vi "Main UI.vi"() -> ()   [LabVIEW 2014]
doc: "This template is for the Queued Message Handler design pattern.\n\nThe Event Handling Loop generates messages based on user interface actions.\n\nThe Message Handling Loop processes messages generated by the Event Handling Loop, or by other messages. The messages are string values, so new messages can be added easily to the Message Cases case structure in the Message Handling Loop. Each message cluster can also provide an optional value for Message Data, which is a variant that can be converted to whatever message-specific data is required."
uses:
  controls/UI Data.ctl
  support/Message Queue/Message Queue.lvlib
  support/User Event - Stop/User Event - Stop.lvlib
panel:
  out "DNL_Data Display <Replace Me>":string
  in  "DNL_Do Something Else <Replace Me>":bool
  in  "DNL_Do Something <Replace Me>":bool
  in  "DNL_Stop Button":bool
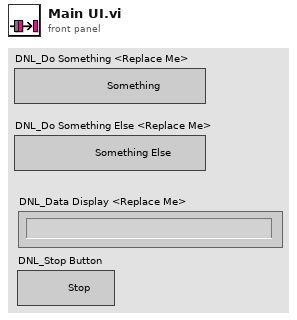
[diagram p1: front panel]
types:
  T1 = typedef "UI Data.ctl" = cluster{"DNL_Boolean <Replace Me>":bool, "DNL_String <Replace Me>":string, "DNL_Numeric <Replace Me>":dbl}
  T2 = typedef "Message Queue.lvlib/All Message Queues.ctl" = cluster{"DNL_UI":refnum<queue>}
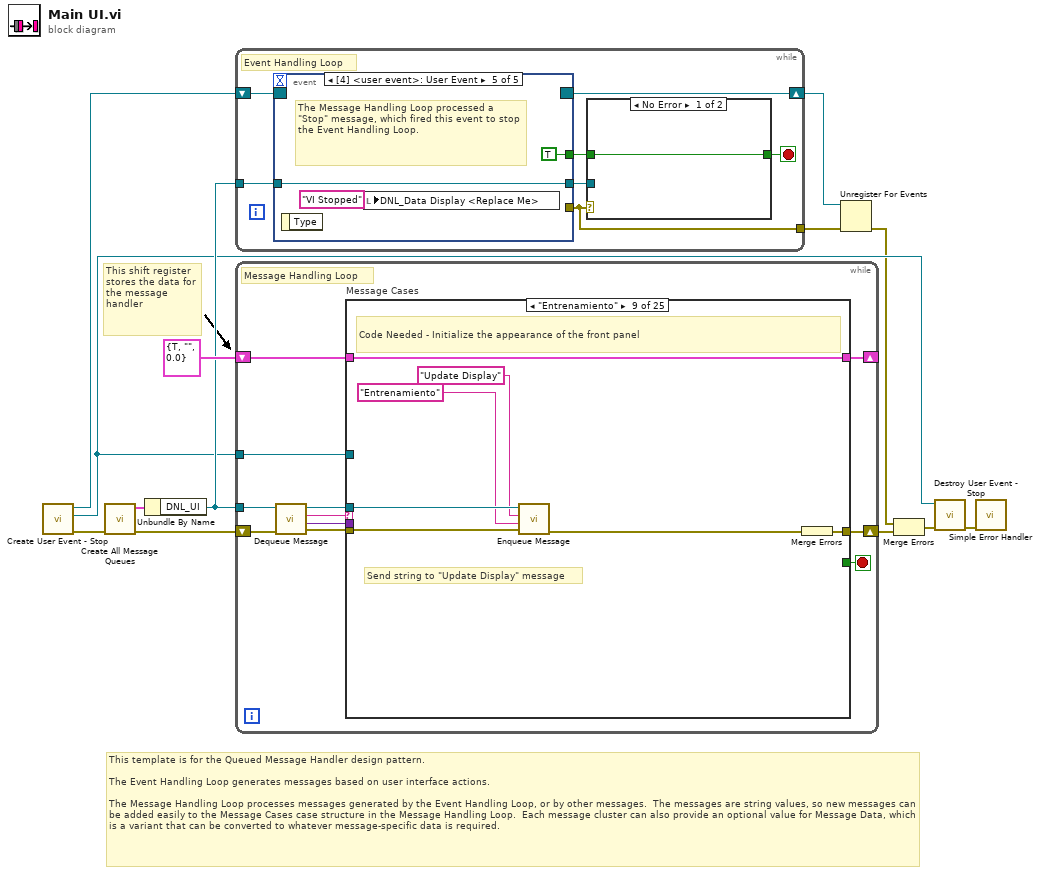
[diagram p0: block diagram]
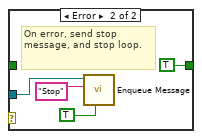
[diagram p2: hidden frame]
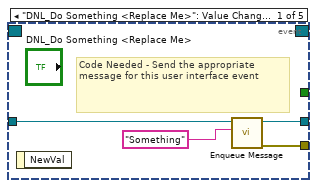
[diagram p3: hidden frame]
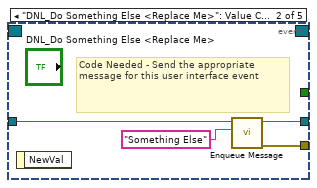
[diagram p4: hidden frame]
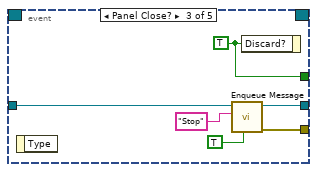
[diagram p5: hidden frame]
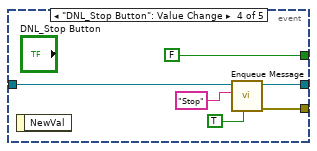
[diagram p6: hidden frame]
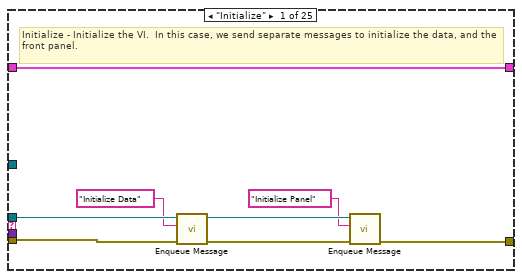
[diagram p7: hidden frame]
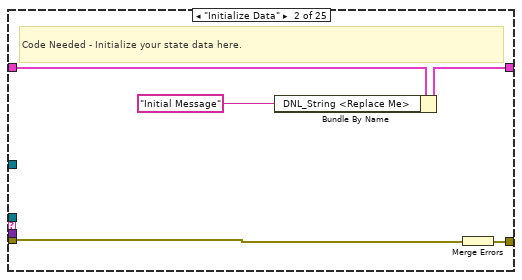
[diagram p8: hidden frame]
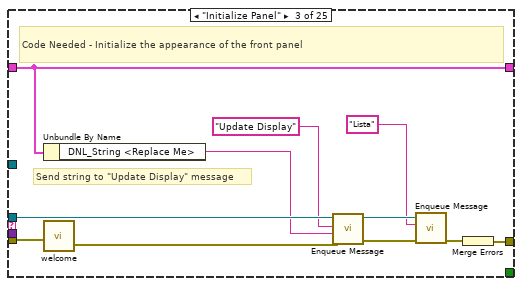
[diagram p9: hidden frame]
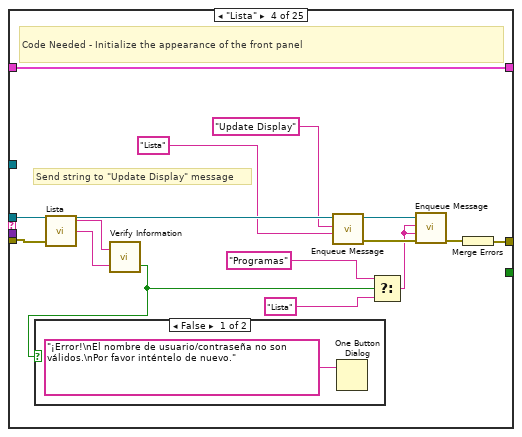
[diagram p10: hidden frame]
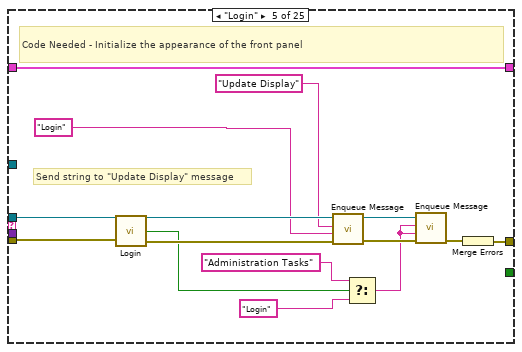
[diagram p12: hidden frame]
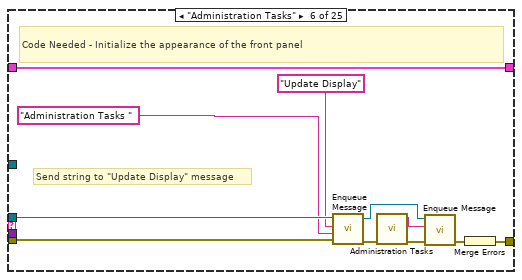
[diagram p13: hidden frame]
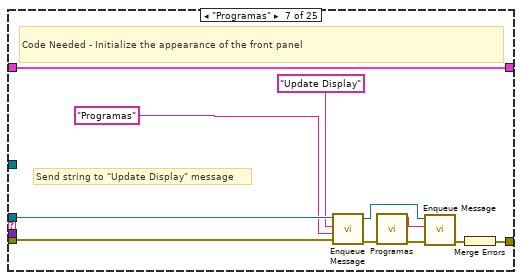
[diagram p14: hidden frame]
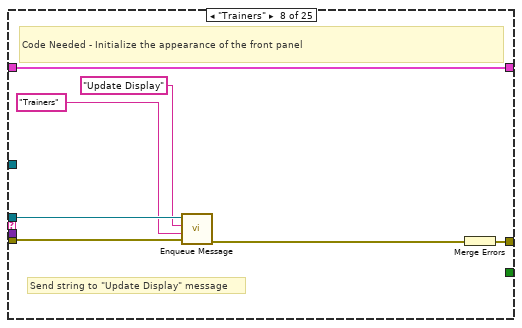
[diagram p15: hidden frame]
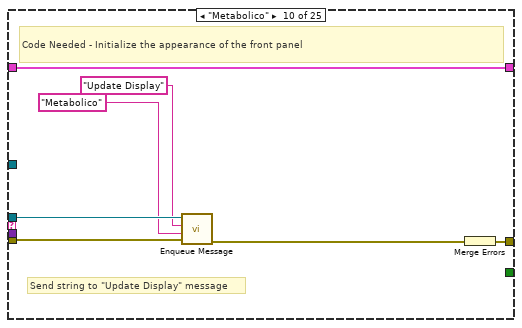
[diagram p16: hidden frame]
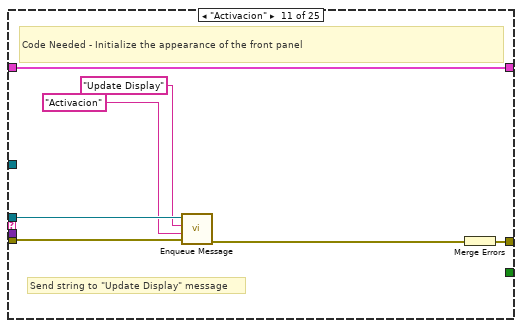
[diagram p17: hidden frame]
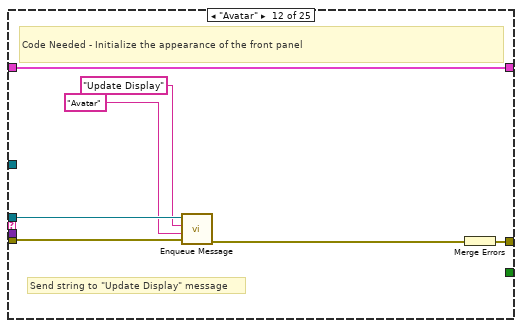
[diagram p18: hidden frame]
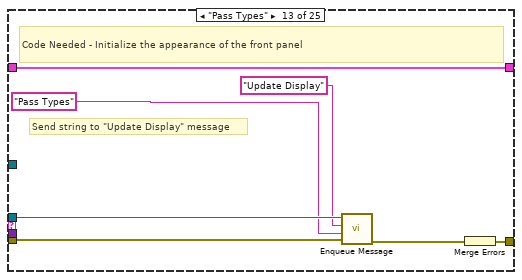
[diagram p19: hidden frame]
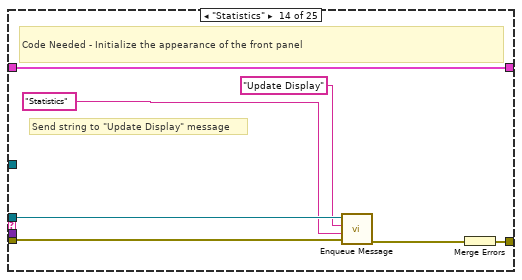
[diagram p20: hidden frame]
diagram:
  # "This template is for the Queued Message Handler design pattern.\n\nThe Event Handling Loop generates messages based on user interface actions.\n\nThe Message Handling Loop processes messages generated by the Event Handling Loop, or by other messages.  The messages are string values, so new messages can be added easily to the Message Cases case structure in the Message Handling Loop.  Each message cluster can also provide an optional value for Message Data, which is a variant that can be converted to whatever message-specific data is required."
  # "This shift register\nstores the data for the message handler"
  n1 = call "Create User Event - Stop.vi"() -> ("error out"=w7:errorcluster, "DNL_User Event - Stop"=w4:refnum<user-event>, "DNL_Stop Event Registration Refnum"=w8:refnum<event-registration>)  [unwired: 9 in]
  n2 = call "Create All Message Queues.vi"("error in (no error)"=w7) -> ("error out"=w13:errorcluster, "DNL_Message Queues out"=w11:T2)  [unwired: 9 in]
  n3 = Unbundle By Name(w11) -> ("DNL_UI"=w9:refnum<queue>)
  n4 = while {
    tunnel: w9 -> [w20]
    tunnel: [w16] -> w2
    shift-right: [w14] -> w1
    shift-left: w8 -> [w15]
    stop <- w18 stop-if-true
    # "Event Handling Loop"
    n5 = event shown="[4] <user event>: User Event" {
      selector: w15 -> [_ _ _ _ _]
      dyn-events: [_ _ _ _ _] -> w14
      timeout: _ -> [_ _ _ _ _]
      tunnel: [_ _ w39 FALSE ("Discard?") TRUE ("Discard?")] -> w19
      tunnel: w20 -> [w29 w33 w38 w45 w48]
      tunnel: [w28 w31 w37 w44 _] -> w16
      tunnel: [w27 w32 w36 w42 w48] -> w17
      event "DNL_Do Something <Replace Me>": Value Change {
        # "Code Needed - Send the appropriate message for this user interface event"
        n6 = event-data() -> ()  [unwired: 1 in, 1 out]
        n7 = call "Enqueue Message.vi"("DNL_Message"="Something" ("Message"), "DNL_Message Queue"=w29) -> ("error out"=w28:errorcluster, "DNL_dup Message Queue"=w27:refnum<queue>)  [unwired: 8 in]
      }
      event "DNL_Do Something Else <Replace Me>": Value Change {
        # "Code Needed - Send the appropriate message for this user interface event"
        n8 = event-data() -> ()  [unwired: 1 in, 1 out]
        n9 = call "Enqueue Message.vi"("DNL_Message"="Something Else" ("Message"), "DNL_Message Queue"=w33) -> ("error out"=w31:errorcluster, "DNL_dup Message Queue"=w32:refnum<queue>)  [unwired: 8 in]
      }
      event Panel Close? {
        w39 = TRUE ("Discard?")
        n10 = event-data() -> ()  [unwired: 1 in, 1 out]
        n11 = call "Enqueue Message.vi"("DNL_Priority Message? (F)"=TRUE ("Priority Message? (F)"), "DNL_Message"="Stop" ("Message"), "DNL_Message Queue"=w38) -> ("error out"=w37:errorcluster, "DNL_dup Message Queue"=w36:refnum<queue>)  [unwired: 7 in]
        n12 = event-data("Discard?"=w39) -> ()  [unwired: 1 in, 1 out]
      }
      event "DNL_Stop Button": Value Change {
        n13 = event-data() -> ()  [unwired: 1 in, 1 out]
        n14 = call "Enqueue Message.vi"("DNL_Priority Message? (F)"=TRUE ("Priority Message? (F)"), "DNL_Message"="Stop" ("Message"), "DNL_Message Queue"=w45) -> ("error out"=w44:errorcluster, "DNL_dup Message Queue"=w42:refnum<queue>)  [unwired: 7 in]
      }
      event User Event {
        # "The Message Handling Loop processed a \"Stop\" message, which fired this event to stop the Event Handling Loop."
        n15 = event-data() -> ()  [unwired: 1 in, 1 out]
        n16 = local write "DNL_Data Display <Replace Me>"("VI Stopped" ("VI Stopped")) -> ()
      }
    }
    n17 = case shown="No Error" w16 {
      tunnel: [w21 TRUE ("Discard?")] -> w18
      tunnel: w19 -> [w21 _]
      tunnel: w17 -> [_ w24]
      frame No Error {
      }
      frame Error {
        # "On error, send stop message, and stop loop."
        n18 = call "Enqueue Message.vi"("DNL_Priority Message? (F)"=TRUE ("Priority Message? (F)"), "DNL_Message"="Stop" ("Message"), "DNL_Message Queue"=w24) -> ()  [unwired: 7 in, 2 out]
      }
    }
  }
  n19 = while {
    tunnel: w9 -> [w49]
    shift-right: [w58] -> _
    shift-left: T1 {"DNL_Boolean <Replace Me>"=TRUE, "DNL_String <Replace Me>"="", "DNL_Numeric <Replace Me>"=0.0} ("Data Cluster") -> [w59]
    tunnel: w4 -> [w55]
    shift-right: [w56] -> w10
    shift-left: w13 -> [w54]
    stop <- w57 stop-if-true
    # "Message Handling Loop"
    n20 = call "Dequeue Message.vi"("error in (no error)"=w54, "DNL_Message Queue"=w49) -> ("error out"=w53:errorcluster, "DNL_Message Data"=w51:variant, "DNL_Message"=w52:string, "DNL_dup Message Queue"=w50:refnum<queue>)  [unwired: 6 in]
    n21 = case "Message Cases" shown="\"Entrenamiento\"" w52 {
      selector: w52 -> [_ _ _ _ _ _ _ _ _ _ _ _ _ _ _ _ _ _ _ _ _ _ _ _ w259]
      tunnel: w50 -> [w62 _ w81 w96 w112 w123 w134 w141 w148 w155 w162 w169 w176 w183 w190 w197 w204 w214 w222 w226 w233 _ _ w255 _]
      tunnel: w53 -> [w65 w72 w78 w90 w107 w121 w132 w139 w146 w153 w160 w167 w174 w181 w188 w195 w202 w212 w220 w228 w235 w242 w247 w250 _]
      tunnel: [w67 w68 w82 w97 w113 w124 w135 w142 w149 w156 w163 w170 w177 w184 w191 w198 w205 w215 w223 w229 w236 w243 w245 w251 w257] -> w56
      tunnel: w59 -> [w66 w71 w83 w98 w101 w115 w126 w137 w144 w151 w158 w165 w172 w179 w186 w193 w200 w211 w219 w230 w237 w244 w246 w254 w261]
      tunnel: [w66 w70 w83 w98 w101 w115 w126 w137 w144 w151 w158 w165 w172 w179 w186 w193 w200 w211 w219 w230 w237 w244 w246 w254 w261] -> w58
      tunnel: [_ _ _ _ _ _ _ _ _ _ _ _ _ _ _ _ _ _ _ _ _ _ _ TRUE _] -> w57
      tunnel: w51 -> [_ _ _ _ _ _ _ _ _ _ _ _ _ _ _ _ _ _ _ _ _ w241 _ _ _]
      tunnel: w55 -> [_ _ _ _ _ _ _ _ _ _ _ _ _ _ _ _ _ _ _ _ _ _ _ w249 _]
      frame "Initialize" {
        # "Initialize - Initialize the VI.  In this case, we send separate messages to initialize the data, and the front panel."
        n22 = call "Enqueue Message.vi"("error in (no error)"=w65, "DNL_Message"="Initialize Data" ("Message"), "DNL_Message Queue"=w62) -> ("error out"=w64:errorcluster, "DNL_dup Message Queue"=w63:refnum<queue>)  [unwired: 7 in]
        n23 = call "Enqueue Message.vi"("error in (no error)"=w64, "DNL_Message"="Initialize Panel" ("Message"), "DNL_Message Queue"=w63) -> ("error out"=w67:errorcluster)  [unwired: 7 in, 1 out]
      }
      frame "Initialize Data" {
        # "Code Needed - Initialize your state data here."
        n24 = Bundle By Name(cluster=w71, "DNL_String <Replace Me>"="Initial Message" ("Initial Message")) -> (w70:T1)
        n25 = Merge Errors(w72) -> (w68:errorcluster)
      }
      frame "Initialize Panel" {
        # "Send string to \"Update Display\" message"
        # "Code Needed - Initialize the appearance of the front panel"
        n26 = Unbundle By Name(w83) -> ("DNL_String <Replace Me>"=w79:string)
        n27 = call "welcome.vi"("error in (no error)"=w78) -> ("error out"=w77:errorcluster)  [unwired: 1 in, 1 out]
        n28 = call "Enqueue Message.vi"("error in (no error)"=w77, "DNL_Message Data"=w79, "DNL_Message"="Update Display" ("Message"), "DNL_Message Queue"=w81) -> ("error out"=w75:errorcluster, "DNL_dup Message Queue"=w74:refnum<queue>)  [unwired: 6 in]
        n29 = call "Enqueue Message.vi"("error in (no error)"=w75, "DNL_Message"="Lista" ("Message"), "DNL_Message Queue"=w74) -> ("error out"=w76:errorcluster)  [unwired: 7 in, 1 out]
        n30 = Merge Errors(w76) -> (w82:errorcluster)
      }
      frame "Lista" {
        # "Send string to \"Update Display\" message"
        # "Code Needed - Initialize the appearance of the front panel"
        n31 = call "Lista.vi"("error in (no error)"=w90) -> ("Password"=w88:string, "Login"=w89:string)  [unwired: 2 in, 1 out]
        n32 = call "Verify Information.vi"("Password"=w88, "User Name"=w89) -> ("Access Granted"=w84:bool)  [unwired: 1 out]
        n33 = case shown="False" w84 {
          frame False {
            n34 = One Button Dialog(message="¡Error!\nEl nombre de usuario/contraseña no son válidos.\nPor favor inténtelo de nuevo.") -> ()  [unwired: 1 in, 1 out]
          }
          frame True {
          }
        }
        n35 = call "Enqueue Message.vi"("DNL_Message Data"="Lista" ("Initial Message"), "DNL_Message"="Update Display" ("Message"), "DNL_Message Queue"=w96) -> ("error out"=w93:errorcluster, "DNL_dup Message Queue"=w92:refnum<queue>)  [unwired: 7 in]
        n36 = Select(t="Programas" ("Message"), s=w84, f="Lista" ("Message")) -> (s? t:f=w85:string)
        n37 = call "Enqueue Message.vi"("error in (no error)"=w93, "DNL_Message Data"=w85, "DNL_Message"=w85, "DNL_Message Queue"=w92) -> ("error out"=w94:errorcluster)  [unwired: 6 in, 1 out]
        n38 = Merge Errors(w94) -> (w97:errorcluster)
      }
      frame "Login" {
        # "Send string to \"Update Display\" message"
        # "Code Needed - Initialize the appearance of the front panel"
        n39 = call "Login.vi"("error in (no error)"=w107) -> ("Access Granted"=w105:bool, "error out"=w106:errorcluster)  [unwired: 1 in, 1 out]
        n40 = call "Enqueue Message.vi"("error in (no error)"=w106, "DNL_Message Data"="Login" ("Initial Message"), "DNL_Message"="Update Display" ("Message"), "DNL_Message Queue"=w112) -> ("error out"=w109:errorcluster, "DNL_dup Message Queue"=w108:refnum<queue>)  [unwired: 6 in]
        n41 = Select(t="Administration Tasks" ("Message"), s=w105, f="Login" ("Message")) -> (s? t:f=w102:string)
        n42 = call "Enqueue Message.vi"("error in (no error)"=w109, "DNL_Message Data"=w102, "DNL_Message"=w102, "DNL_Message Queue"=w108) -> ("error out"=w110:errorcluster)  [unwired: 6 in, 1 out]
        n43 = Merge Errors(w110) -> (w113:errorcluster)
      }
      frame "Administration Tasks" {
        # "Send string to \"Update Display\" message"
        # "Code Needed - Initialize the appearance of the front panel"
        n44 = call "Enqueue Message.vi"("error in (no error)"=w121, "DNL_Message Data"="Administration Tasks " ("Initial Message"), "DNL_Message"="Update Display" ("Message"), "DNL_Message Queue"=w123) -> ("error out"=w120:errorcluster, "DNL_dup Message Queue"=w116:refnum<queue>)  [unwired: 6 in]
        n45 = call "Administration Tasks.vi"("error in (no error)"=w120) -> ("error out"=w119:errorcluster, "Message"=w117:string)  [unwired: 9 in]
        n46 = call "Enqueue Message.vi"("error in (no error)"=w119, "DNL_Message"=w117, "DNL_Message Queue"=w116) -> ("error out"=w118:errorcluster)  [unwired: 7 in, 1 out]
        n47 = Merge Errors(w118) -> (w124:errorcluster)
      }
      frame "Programas" {
        # "Send string to \"Update Display\" message"
        # "Code Needed - Initialize the appearance of the front panel"
        n48 = call "Enqueue Message.vi"("error in (no error)"=w132, "DNL_Message Data"="Programas" ("Initial Message"), "DNL_Message"="Update Display" ("Message"), "DNL_Message Queue"=w134) -> ("error out"=w131:errorcluster, "DNL_dup Message Queue"=w127:refnum<queue>)  [unwired: 6 in]
        n49 = call "Programas.vi"("error in (no error)"=w131) -> ("error out"=w130:errorcluster, "Message"=w128:string)  [unwired: 9 in]
        n50 = call "Enqueue Message.vi"("error in (no error)"=w130, "DNL_Message"=w128, "DNL_Message Queue"=w127) -> ("error out"=w129:errorcluster)  [unwired: 7 in, 1 out]
        n51 = Merge Errors(w129) -> (w135:errorcluster)
      }
      frame "Trainers" {
        # "Send string to \"Update Display\" message"
        # "Code Needed - Initialize the appearance of the front panel"
        n52 = call "Enqueue Message.vi"("error in (no error)"=w139, "DNL_Message Data"="Trainers" ("Initial Message"), "DNL_Message"="Update Display" ("Message"), "DNL_Message Queue"=w141) -> ("error out"=w138:errorcluster)  [unwired: 6 in, 1 out]
        n53 = Merge Errors(w138) -> (w142:errorcluster)
      }
      frame "Entrenamiento" {
        # "Send string to \"Update Display\" message"
        # "Code Needed - Initialize the appearance of the front panel"
        n54 = call "Enqueue Message.vi"("error in (no error)"=w146, "DNL_Message Data"="Entrenamiento" ("Initial Message"), "DNL_Message"="Update Display" ("Message"), "DNL_Message Queue"=w148) -> ("error out"=w145:errorcluster)  [unwired: 6 in, 1 out]
        n55 = Merge Errors(w145) -> (w149:errorcluster)
      }
      frame "Metabolico" {
        # "Send string to \"Update Display\" message"
        # "Code Needed - Initialize the appearance of the front panel"
        n56 = call "Enqueue Message.vi"("error in (no error)"=w153, "DNL_Message Data"="Metabolico" ("Initial Message"), "DNL_Message"="Update Display" ("Message"), "DNL_Message Queue"=w155) -> ("error out"=w152:errorcluster)  [unwired: 6 in, 1 out]
        n57 = Merge Errors(w152) -> (w156:errorcluster)
      }
      frame "Activacion" {
        # "Send string to \"Update Display\" message"
        # "Code Needed - Initialize the appearance of the front panel"
        n58 = call "Enqueue Message.vi"("error in (no error)"=w160, "DNL_Message Data"="Activacion" ("Initial Message"), "DNL_Message"="Update Display" ("Message"), "DNL_Message Queue"=w162) -> ("error out"=w159:errorcluster)  [unwired: 6 in, 1 out]
        n59 = Merge Errors(w159) -> (w163:errorcluster)
      }
      frame "Avatar" {
        # "Send string to \"Update Display\" message"
        # "Code Needed - Initialize the appearance of the front panel"
        n60 = call "Enqueue Message.vi"("error in (no error)"=w167, "DNL_Message Data"="Avatar" ("Initial Message"), "DNL_Message"="Update Display" ("Message"), "DNL_Message Queue"=w169) -> ("error out"=w166:errorcluster)  [unwired: 6 in, 1 out]
        n61 = Merge Errors(w166) -> (w170:errorcluster)
      }
      frame "Pass Types" {
        # "Send string to \"Update Display\" message"
        # "Code Needed - Initialize the appearance of the front panel"
        n62 = call "Enqueue Message.vi"("error in (no error)"=w174, "DNL_Message Data"="Pass Types" ("Initial Message"), "DNL_Message"="Update Display" ("Message"), "DNL_Message Queue"=w176) -> ("error out"=w173:errorcluster)  [unwired: 6 in, 1 out]
        n63 = Merge Errors(w173) -> (w177:errorcluster)
      }
      frame "Statistics" {
        # "Send string to \"Update Display\" message"
        # "Code Needed - Initialize the appearance of the front panel"
        n64 = call "Enqueue Message.vi"("error in (no error)"=w181, "DNL_Message Data"="Statistics" ("Initial Message"), "DNL_Message"="Update Display" ("Message"), "DNL_Message Queue"=w183) -> ("error out"=w180:errorcluster)  [unwired: 6 in, 1 out]
        n65 = Merge Errors(w180) -> (w184:errorcluster)
      }
      frame "Languages" {
        # "Send string to \"Update Display\" message"
        # "Code Needed - Initialize the appearance of the front panel"
        n66 = call "Enqueue Message.vi"("error in (no error)"=w188, "DNL_Message Data"="Languages" ("Initial Message"), "DNL_Message"="Update Display" ("Message"), "DNL_Message Queue"=w190) -> ("error out"=w187:errorcluster)  [unwired: 6 in, 1 out]
        n67 = Merge Errors(w187) -> (w191:errorcluster)
      }
      frame "Date Time" {
        # "Send string to \"Update Display\" message"
        # "Code Needed - Initialize the appearance of the front panel"
        n68 = call "Enqueue Message.vi"("error in (no error)"=w195, "DNL_Message Data"="Date Time" ("Initial Message"), "DNL_Message"="Update Display" ("Message"), "DNL_Message Queue"=w197) -> ("error out"=w194:errorcluster)  [unwired: 6 in, 1 out]
        n69 = Merge Errors(w194) -> (w198:errorcluster)
      }
      frame "Back" {
        # "Send string to \"Update Display\" message"
        # "Code Needed - Initialize the appearance of the front panel"
        n70 = call "Enqueue Message.vi"("error in (no error)"=w202, "DNL_Message Data"="Back" ("Initial Message"), "DNL_Message"="Update Display" ("Message"), "DNL_Message Queue"=w204) -> ("error out"=w201:errorcluster)  [unwired: 6 in, 1 out]
        n71 = Merge Errors(w201) -> (w205:errorcluster)
      }
      frame "Reset" {
        # "Send string to \"Update Display\" message"
        # "Code Needed - Initialize the appearance of the front panel"
        n72 = call "Enqueue Message.vi"("error in (no error)"=w212, "DNL_Message Data"="Reset" ("Initial Message"), "DNL_Message"="Update Display" ("Message"), "DNL_Message Queue"=w214) -> ("error out"=w209:errorcluster, "DNL_dup Message Queue"=w207:refnum<queue>)  [unwired: 6 in]
        n73 = call "Enqueue Message.vi"("error in (no error)"=w209, "DNL_Message"="Initialize" ("Message"), "DNL_Message Queue"=w207) -> ("error out"=w208:errorcluster)  [unwired: 7 in, 1 out]
        n74 = Merge Errors(w208) -> (w215:errorcluster)
      }
      frame "Help" {
        # "Send string to \"Update Display\" message"
        # "Code Needed - Initialize the appearance of the front panel"
        n75 = call "Enqueue Message.vi"("error in (no error)"=w220, "DNL_Message Data"="Help" ("Initial Message"), "DNL_Message"="Update Display" ("Message"), "DNL_Message Queue"=w222) -> ("error out"=w217:errorcluster)  [unwired: 6 in, 1 out]
        n76 = call "Help.vi"("error in (no error)"=w217) -> ("error out"=w218:errorcluster)  [unwired: 10 in]
        n77 = Merge Errors(w218) -> (w223:errorcluster)
      }
      frame "Something" {
        # "Send string to \"Update Display\" message"
        # "Code Needed - Perform whatever actions correspond to the \"Something\" message"
        n78 = call "Enqueue Message.vi"("error in (no error)"=w228, "DNL_Message Data"="\"Do Something\" button pressed" ("\"Do Something\" button pressed"), "DNL_Message"="Update Display" ("Message"), "DNL_Message Queue"=w226) -> ("error out"=w227:errorcluster)  [unwired: 6 in, 1 out]
        n79 = Merge Errors(w227) -> (w229:errorcluster)
      }
      frame "Something Else" {
        # "Send string to \"Update Display\" message"
        # "Code Needed - Perform whatever actions correspond to the \"Something Else\" message"
        n80 = call "Enqueue Message.vi"("error in (no error)"=w235, "DNL_Message Data"="\"Do Something Else\" button pressed" ("\"Do Something Else\" button pressed"), "DNL_Message"="Update Display" ("Message"), "DNL_Message Queue"=w233) -> ("error out"=w234:errorcluster)  [unwired: 6 in, 1 out]
        n81 = Merge Errors(w234) -> (w236:errorcluster)
      }
      frame "Update Display" {
        # "Code Recommended - If you wish to decouple the Message Handling Loop from your user interface, consider creating User Events (like the \"Stop\" event in this VI) to message the Event Handling Loop whenever the user interface needs updating."
        # "Update Display - Convert the message data to a string to display in the Data Display indicator."
        n82 = Variant To Data(error in=w242, type="", Variant=w241) -> (data=→"DNL_Data Display <Replace Me>":string, error out=w239:errorcluster)
        n83 = Merge Errors(w239) -> (w243:errorcluster)
      }
      frame "---Copy This Frame---" {
        # "Duplicate this frame when creating new messages.  Change this comment in the duplicated frame to describe this message."
        n84 = Merge Errors(w247) -> (w245:errorcluster)
      }
      frame "Stop" {
        # "Stop the VI"
        # "Release the message queue reference"
        # "Code Needed - Add any required cleanup code here"
        n85 = call "Fire User Event - Stop.vi"("DNL_User Event - Stop"=w249) -> ("error out"=w248:errorcluster)  [unwired: 10 in]
        n86 = Release Queue(queue=w255, error in (no error)=w250) -> (error out=w252:errorcluster)  [unwired: 1 in, 2 out]
        n87 = Merge Errors(w248, w252) -> (w251:errorcluster)
      }
      frame Default {
        # "'Default' case only runs if there is a message that isn't defined in any of the other cases.  Output a programming error."
        n88 = Format Into String(format string="The invalid message string \"%s\" was received in the Message Handling Loop." ("Unknown Message Error Text"), w259) -> (resulting string=w256:string)  [unwired: 2 in, 1 out]
        n89 = call <vilib>:"Error Cluster From Error Code.vi"("error message (\"\")"=w256, "error code (0)"=1) -> ("error out"=w257:errorcluster)  [unwired: 7 in]
      }
    }
  }
  n90 = Unregister For Events(event registration refnum=w1, error in=w2) -> (error out=w3:errorcluster)
  n91 = Merge Errors(w3, w10) -> (w5:errorcluster)
  n92 = call "Destroy User Event - Stop.vi"("error in (no error)"=w5, "DNL_User Event - Stop"=w4) -> ("error out"=w6:errorcluster)  [unwired: 9 in]
  n93 = call <vilib>:"Simple Error Handler.vi"("error in (no error)"=w6) -> ()  [unwired: 4 in, 5 out]
